vi "Adresse UsrVal.vi"(8 "error in (no error)":errorcluster caption="Fehler (Eingang, kein Fehler)", 11 "Steuerung PNS Eingang":refnum<class "Steuerung PNS.lvclass">) -> (0 "error out":errorcluster caption="Fehler (Ausgang)", 2 "Adressen":T1, 3 "Steuerung PNS Ausgang":refnum<class "Steuerung PNS.lvclass">)   [LabVIEW 2020, in "Steuerung PNS.lvclass"]
uses:
  Steuerung PNS.lvclass
  Adresse.ctl
  AdressIndex.ctl
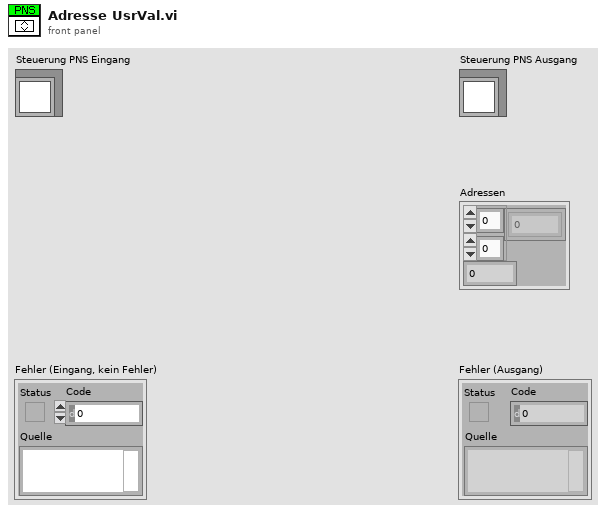
[diagram p1: front panel]
types:
  T1 = typedef "Steuerung PNS.lvclass/Adresse.ctl" = cluster{i32[][], i32}
  T2 = typedef "Steuerung PNS.lvclass/AdressIndex.ctl" = cluster{"Index":i32, "Index 2":i32, "Länge2":i32, "\nAnzahl":i32}
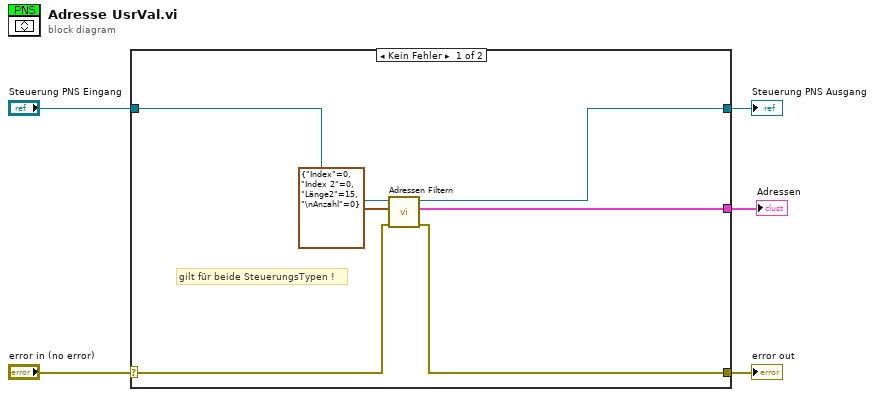
[diagram p0: block diagram]
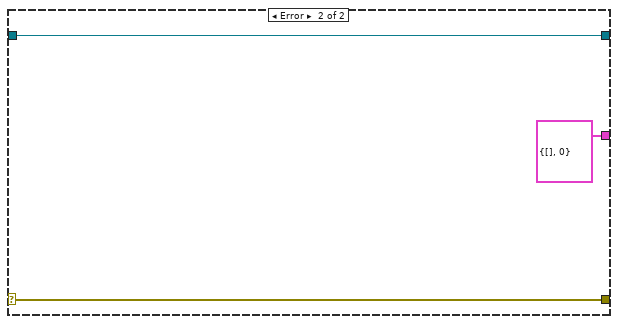
[diagram p2: hidden frame]
diagram:
  n1 = case shown="Kein Fehler" "error in (no error)" {
    selector: "error in (no error)" -> [w10 w14]
    tunnel: [w9 w14] -> w4
    tunnel: [w6 w13] -> w2
    tunnel: "Steuerung PNS Eingang" -> [w7 w13]
    tunnel: [w8 T1 {[], 0} ("Adressen")] -> w1
    frame No Error {
      # "gilt für beide SteuerungsTypen !"
      n2 = call "Adressen Filtern.vi"("error in (no error)"=w10, "AdressIndex"=T2 {"Index"=0, "Index 2"=0, "Länge2"=15, "\nAnzahl"=0}, "Steuerung PNS Eingang"=w7) -> ("error out"=w9:errorcluster, "Adressen"=w8:cluster{i32[][], i32}, "Steuerung PNS Ausgang"=w6:refnum<class "Steuerung PNS.lvclass">)  [unwired: 6 in]
    }
    frame Error {
    }
  }
  "error out" <- w4
  "Steuerung PNS Ausgang" <- w2
  "Adressen" <- w1
